vi "Wait.vi"(8 "error in (no error)":errorcluster, 11 "User Interface Handler in":refnum<class "User Interface Handler.lvclass">) -> (0 "error out":errorcluster, 2 "User Interface":refnum<class "User Interface.lvclass">, 3 "User Interface Handler out":refnum<class "User Interface Handler.lvclass">)   [LabVIEW 2019, in "DSF Core.lvlib" / "User Interface Handler.lvclass"]
uses:
  User Interface Handler.lvclass
  User Interface/User Interface.lvclass
  User Interface Handler.lvclass/User Interface Handler.ctl
  User Interface Ref.ctl
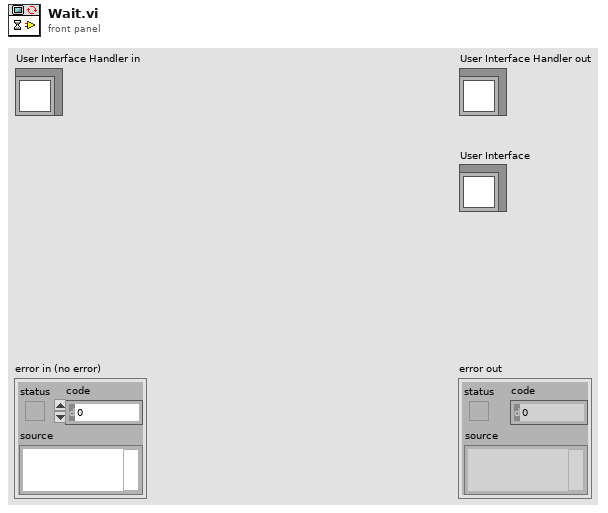
[diagram p1: front panel]
types:
  T1 = typedef "DSF Core.lvlib/User Interface Handler.lvclass/User Interface Ref.ctl" = refnum<vi>
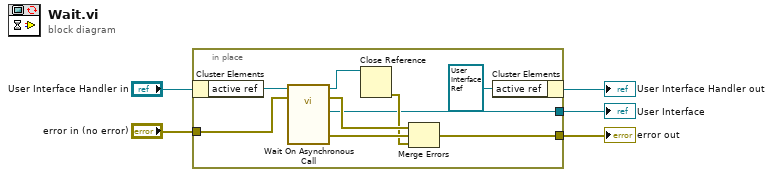
[diagram p0: block diagram]
diagram:
  n1 = in-place {
    in-place-border: [w7] -> w1
    in-place-border: [w12] -> w2
    in-place-border: "error in (no error)" -> [w11]
    n2 = in-place-cluster #1("User Interface Handler in") -> ("active ref"=w14:T1)
    n3 = call-by-ref "Wait On Asynchronous Call"(reference=w14, error in=w11) -> (reference out=w10:T1, error out=w13:errorcluster, 0:"error out"=w9:errorcluster, "User Interface out"=w7:refnum<class "User Interface.lvclass">)  [unwired: 10 in]
    n4 = Close Reference(reference=w10) -> (error out=w8:errorcluster)  [unwired: 1 in]
    n5 = Merge Errors(w13, w9, w8) -> (w12:errorcluster)
    n6 = in-place-cluster #1("active ref"=T1 refnum) -> (→"User Interface Handler out":refnum<class "User Interface Handler.lvclass">)
  }
  "error out" <- w2
  "User Interface" <- w1
